vi "fgv_Bcknd MovCor window open.vi"(8 "error in (no error)":errorcluster, 9 "Function":T1, 11 "Background MovCor window is open":bool) -> (0 "error out":errorcluster, 3 "Background MovCor window is open":bool)   [LabVIEW 2020]
uses:
  Typedefs/Read Write Enum.ctl
panel:
  # "SUBROUTINE"
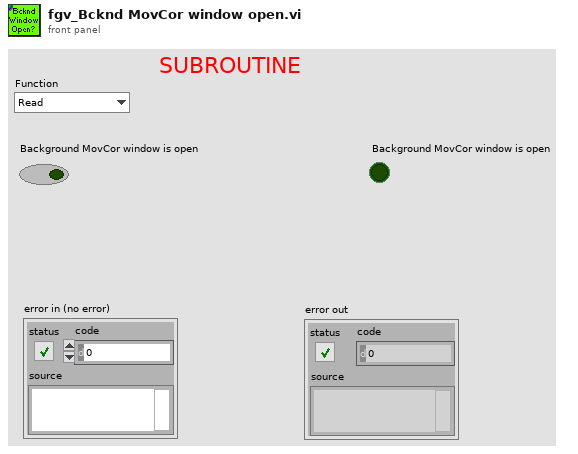
[diagram p1: front panel]
types:
  T1 = typedef "Read Write Enum.ctl" = enum16{"Read", "Write"}
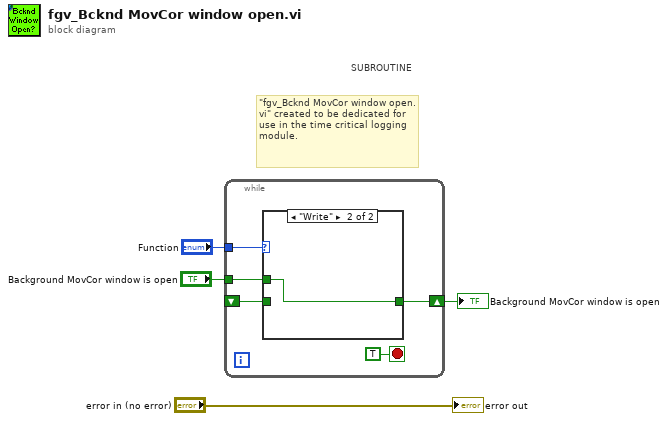
[diagram p0: block diagram]
diagram:
  # "\"fgv_Bcknd MovCor window open.vi\" created to be dedicated for use in the time critical logging module."
  # "SUBROUTINE"
  n1 = while {
    tunnel: "Function" -> [w8]
    tunnel: "Background MovCor window is open" -> [w7]
    shift-right: [w6] -> w2
    shift-left: _ -> [w5]
    stop <- TRUE stop-if-true
    n2 = case shown="\"Write\"" w8 {
      tunnel: w7 -> [_ w11]
      tunnel: [w10 w11] -> w6
      tunnel: w5 -> [w10 _]
      frame "Read", Default {
      }
      frame "Write" {
      }
    }
  }
  "Background MovCor window is open" <- w2
  "error out" <- "error in (no error)"
